vi "YRDParaRead.vi"(11 "字符串":string) -> (0 "错误输出":errorcluster, 1 "SetPressure":dbl, 2 "SetDif":dbl, 3 "引用句柄输出":T1 caption="refnum out", 4 "SetVol":dbl, 5 "SafePre":dbl)   [LabVIEW 2014]
uses:
  <vilib>/Utility/config.llb/Config Data RefNum.ctl
  <vilib>/Utility/config.llb/Read Key (Double).vi
  <vilib>/Utility/config.llb/NI_LVConfig.lvlib
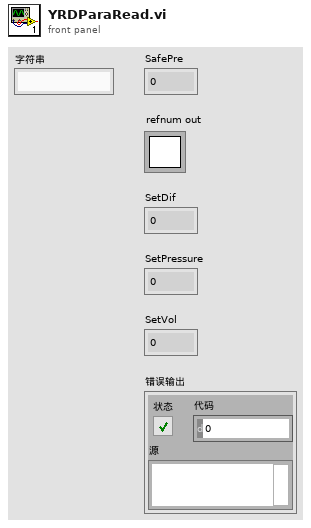
[diagram p1: front panel]
types:
  T1 = typedef "NI_LVConfig.lvlib/Config Data RefNum.ctl" = refnum<k1>
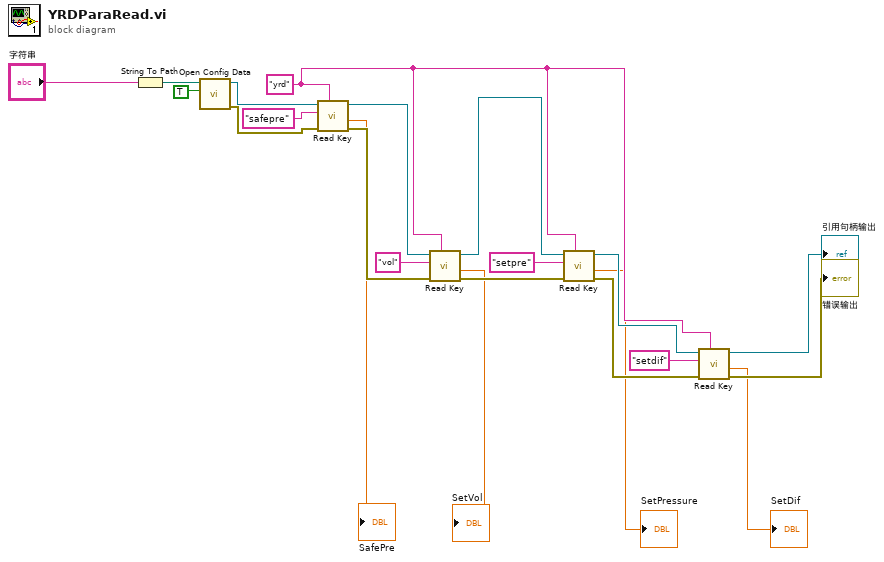
[diagram p0: block diagram]
diagram:
  w18 = "yrd" ("section")
  n1 = String To Path(string="字符串") -> (path=w2:path)
  n2 = call <vilib>:"Open Config Data.vi"("create file if necessary (T)"=TRUE, "configuration file path"=w2) -> ("error out"=w11:errorcluster, "refnum"=w4:T1)  [unwired: 1 in, 7 out]
  n3 = call-poly <vilib>:"Read Key.vi"("section"=w18, "error in (no error)"=w11, "key"="safepre", "refnum"=w4) -> ("error out"=w10:errorcluster, "value"=→"SafePre":dbl, "refnum out"=w7:T1)  [unwired: 4 in, 1 out]
  n4 = call-poly <vilib>:"Read Key.vi"("section"=w18, "error in (no error)"=w10, "key"="vol", "refnum"=w7) -> ("error out"=w22:errorcluster, "value"=→"SetVol":dbl, "refnum out"=w12:T1)  [unwired: 4 in, 1 out]
  n5 = call-poly <vilib>:"Read Key.vi"("section"=w18, "error in (no error)"=w22, "key"="setpre", "refnum"=w12) -> ("error out"=w21:errorcluster, "value"=→"SetPressure":dbl, "refnum out"=w15:T1)  [unwired: 4 in, 1 out]
  n6 = call-poly <vilib>:"Read Key.vi"("section"=w18, "error in (no error)"=w21, "key"="setdif", "refnum"=w15) -> ("error out"=→"错误输出":errorcluster, "value"=→"SetDif":dbl, "refnum out"=→"引用句柄输出":T1)  [unwired: 4 in, 1 out]
